vi "test_find_consecutive_close_values.vi"() -> ()   [LabVIEW 2024]
uses:
  <vilib>/Utility/file.llb/Read Delimited Spreadsheet (string).vi
panel:
  out "#elements found":i32
  out "average":dbl
  in  "csv_data_file_name":string(combo)="low-1.csv"
  in  "python_module_name":string="find_consecutive_close_values.py"
  out "Measures Plot":dbl[][](graph)
  out "data qty":i32
  out "close values":dbl[](array[numeric])
  in  "tolerance%":dbl(slide)=2.0 min=0.0 scale=0.0..10.0
  in  "min_threshold [W]":dbl(slide)=25.0 min=0.0 scale=0.0..100.0
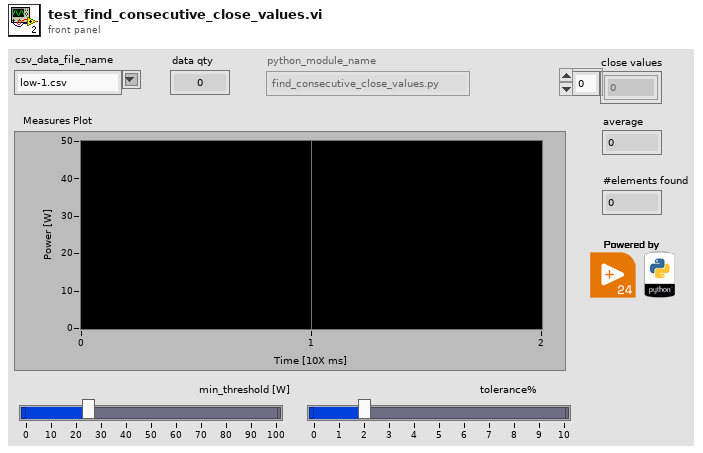
[diagram p1: front panel]
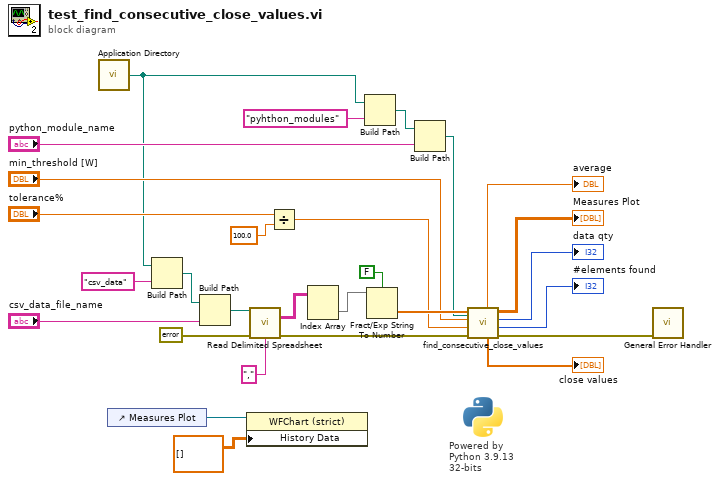
[diagram p0: block diagram]
diagram:
  # "Powered by \nPython 3.9.13\n32-bits"
  n1 = call <vilib>:"Application Directory.vi"() -> ("Application Directory"=w1:path)
  n2 = control-ref of="Measures Plot"() -> (w21:refnum<vi>)
  n3 = Build Path(base path=w1, name or relative path="csv_data") -> (appended path=w17:path)
  n4 = Build Path(base path=w17, name or relative path="csv_data_file_name") -> (appended path=w14:path)
  n5 = property class="WFChart (strict)"(reference=w21, "History Data"=dbl[][] []) -> ()  [unwired: 1 in, 2 out]
  n6 = call-poly <vilib>:"Read Delimited Spreadsheet.vi"("file path (dialog if empty)"=w14, "error in (no error)"=errorcluster {"status"=FALSE, "code"=0, "source"=""} ("error constant"), "delimiter (\\t)"=",") -> ("all rows"=w26:string[][], "error out"=w4:errorcluster)  [unwired: 7 in, 4 out]
  n7 = Divide(x="tolerance%", y=100.0) -> (x/y=w6:dbl)
  n8 = Index Array(array=w26) -> (element=w24:string[])  [unwired: 2 in]
  n9 = Build Path(base path=w1, name or relative path="pyhthon_modules") -> (appended path=w18:path)
  n10 = Fract/Exp String To Number(use system decimal point (T)=FALSE, string=w24) -> (number=w28:dbl[])  [unwired: 2 in, 1 out]
  n11 = Build Path(base path=w18, name or relative path="python_module_name") -> (appended path=w11:path)
  n12 = call "find_consecutive_close_values.vi"("module path"=w11, "error in (no error)"=w4, "tolerance"=w6, "min_threshold"="min_threshold [W]", "data"=w28) -> ("error out"=w3:errorcluster, "#_elements_found"=→"#elements found":i32, "data qty"=→"data qty":i32, "Measures"=→"Measures Plot":dbl[][], "close_values"=→"close values":dbl[], "average"=→"average":dbl)  [unwired: 1 in]
  n13 = call <vilib>:"General Error Handler.vi"("error in (no error)"=w3) -> ()  [unwired: 10 in, 5 out]
